vi "BuildParamsMsg.vi"(0 "Parameters":cluster{"Joint":string, "value":dbl}[](array[cluster])) -> (1 "left msg":string, 2 "right msg":string)   [LabVIEW 2010]
uses:
  <userlib>/ROSforLV_0.1/ROS/MessageBuilding/Primitives/subs/float64Array.vi
  <userlib>/ROSforLV_0.1/ROS/MessageBuilding/Primitives/subs/stringArray.vi
panel:
  in  "Joints":T1(ring)
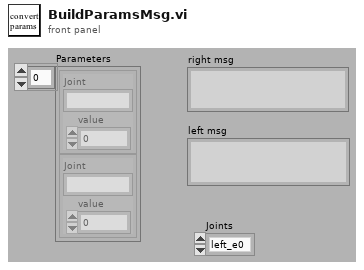
[diagram p1: front panel]
types:
  T1 = enum16{"left_e0", "left_e1", "left_s0", "left_s1", "left_w0", "left_w1", "left_w2", "right_e0", "right_e1", "right_s0", "right_s1", "right_w0", "right_w1", "right_w2"}
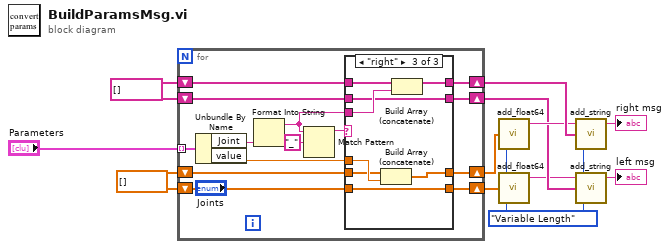
[diagram p0: block diagram]
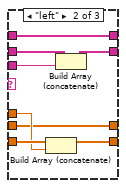
[diagram p3: hidden frame]
diagram:
  w10 = enum16{"Fixed Length", "Variable Length"}."Variable Length" ("Array Type")
  w5 = dbl[] []
  w6 = string[] []
  n1 = for {
    shift-right: [w23] -> w3
    shift-left: w6 -> [w26]
    shift-right: [w24] -> w4
    shift-left: w5 -> [w25]
    tunnel: "Parameters" -> [w22] mode=indexing
    shift-right: [w15] -> w9
    shift-left: w6 -> [w16]
    shift-right: [w13] -> w8
    shift-left: w5 -> [w14]
    n2 = Unbundle By Name(w22) -> ("Joint"=w19:string, "value"=w21:dbl)
    n3 = Format Into String(w19) -> (resulting string=w20:string)  [unwired: 3 in, 1 out]
    n4 = Match Pattern(string=w20, regular expression="_") -> (before substring=w17:string)  [unwired: 1 in, 3 out]
    n5 = case shown="\"right\"" w17 {
      tunnel: w26 -> [w30 w38 w42]
      tunnel: w25 -> [w29 w36 w39]
      tunnel: [w29 w35 w39] -> w24
      tunnel: [w30 w37 w42] -> w23
      tunnel: w21 -> [_ w34 w46]
      tunnel: w20 -> [_ w33 w45]
      tunnel: w16 -> [w28 w32 w44]
      tunnel: [w28 w32 w43] -> w15
      tunnel: w14 -> [w27 w31 w41]
      tunnel: [w27 w31 w40] -> w13
      frame Default {
      }
      frame "left" {
        n6 = Build Array (concatenate)(w36, w34) -> (w35:dbl[])
        n7 = Build Array (concatenate)(w38, w33) -> (w37:string[])
      }
      frame "right" {
        n8 = Build Array (concatenate)(w41, w46) -> (w40:dbl[])
        n9 = Build Array (concatenate)(w44, w45) -> (w43:string[])
      }
    }
  }
  n10 = call-poly <userlib>:"add_float64.vi"("Array Type"=w10, "Array"=w8) -> ("msg out"=w7:string)  [unwired: 3 in]
  n11 = call-poly <userlib>:"add_float64.vi"("Array Type"=w10, "Array"=w4) -> ("msg out"=w2:string)  [unwired: 3 in]
  n12 = call-poly <userlib>:"add_string.vi"("Array Type"=w10, "Array"=w9, "msg in"=w7) -> ("msg out"=→"right msg":string)  [unwired: 2 in]
  n13 = call-poly <userlib>:"add_string.vi"("Array Type"=w10, "Array"=w3, "msg in"=w2) -> ("msg out"=→"left msg":string)  [unwired: 2 in]
